vi "Cache.CheckStatus.vi"(7 "Idx":i32, 8 "error in":errorcluster, 10 "CheckStatus in":T5, 11 "Data in":T1) -> (0 "error out":errorcluster, 2 "CheckStatus out":T4, 3 "Data out":T1)   [LabVIEW 2016]
doc: "Write test results (measurement values) to proda database\n\nWabco 2017 All right reserved\nAuthor: maciej.szupienko@wabco-auto.com"
uses:
  Drivers/PLC/LowLevel/PLC.DataBlock.PLCcheckstatus.ctl
  Drivers/PLC/LowLevel/PLC.DataBlock.PCcheckstatus.ctl
  Cache.Data.ctl
  Cache.Data.Status.ctl
  Cache.Data.Sets.ctl
  Cache.ProductComponent.Data.ctl
  Tools/EventLog/EventLog.EventSource.ctl
  Tools/EventLog/EventLog.EventLevel.ctl
  Tools/Translator/Translator.Message.ctl
  Tools/EventLog/EventLog.New(array).vi
  Global/ApplicationGlobal.vi
  Tools/EventLog/EventLog.Buffer.vi
  Tools/EventLog/EventLog.File.ReadWrite.vi
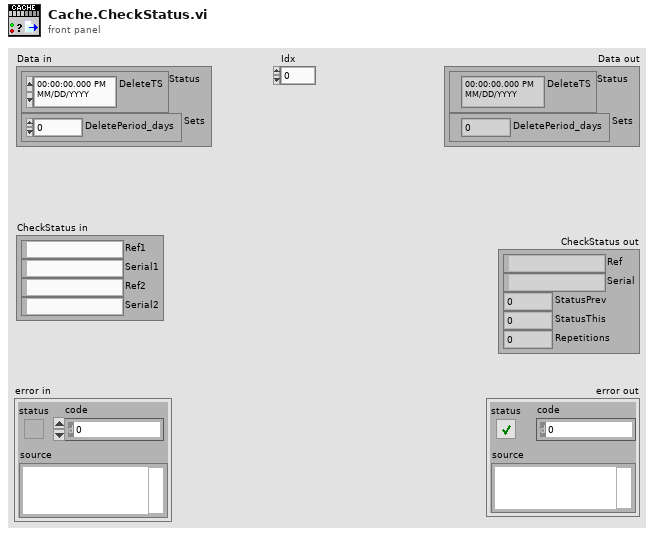
[diagram p1: front panel]
types:
  T1 = typedef "Cache.Data.ctl" = cluster{"Status":T2, "Sets":T3}
  T2 = typedef "Cache.Data.Status.ctl" = cluster{"DeleteTS":timestamp}
  T3 = typedef "Cache.Data.Sets.ctl" = cluster{"DeletePeriod_days":dbl}
  T4 = typedef "PLC.DataBlock.PCcheckstatus.ctl" = cluster{"Ref":string, "Serial":string, "StatusPrev":i8, "StatusThis":i8, "Repetitions":u8}
  T5 = typedef "PLC.DataBlock.PLCcheckstatus.ctl" = cluster{"Ref1":string, "Serial1":string, "Ref2":string, "Serial2":string}
  T6 = typedef "EventLog.EventSource.ctl" = enum16{"All", "Gui", "Cache", "PLC1", "PLC2", "PLC3", "DB", "DB01", "DB02", "DB03", "DB04", "DB05", "DB06", "DB07", "DB08", "DB09", "DB10", "DB11", "DB12", "DB13", "DB14", "DB15", "DB16"}
  T7 = typedef "Cache.ProductComponent.Data.ctl" = cluster{"Time":timestamp, "Station":string, "Ref1":string, "Serial1":string, "Ref2":string, "Serial2":string}
  T8 = typedef "Translator.Message.ctl" = enum16{"-", "Event confirmed", "Log out", "Log in", "Shutdown", "Cancel", "Start", "Continue", "Stop", "On", "Off", "OK", "NOK", "NOK %s", "This", "Prev", "Home", "Work", "In progress...", "Missing", "Empty", "Hardware failure", "Initial", "Error %d >> %s", "Error %d >> %s >> %s", "Starting %s", "Quitting %s", "Configured", "Initializing", "Quitting", "Loading", "Running %s", "Stopped", "Summary", "Do you want to continue?", "Do you want to exit?", "Log out?", "System", "All", "IDLE", "Translating...%s", "Not found", "Alarm %s", "Run", "Skip", "Abort", "Repeat", "Please wait...", "Database disconnected", "Login to database successful", "Login to database failed: %d; %s", "Get process step data for %s", "Changeover off", "Changeover into %s", "Product %s | %s found in cache with status %d at previous station", "Product %s | %s found in database with status %d at previous station", "Product %s | %s not found in cache at previous station", "Product %s | %s not found in database at previous station", "Product %s | %s found in cache with status %d at this station (%d repetion)", "Product %s | %s found in database with status %d at this station (%d repetition)", "Product %s | %s not found in cache at this station", "Product %s | %s not found in database at this station", "Product %s | %s found in cache for component %s | %s", "Product %s | %s found in database for component %s | %s", "Product not found in cache for component %s | %s", "Product not found in database for component %s | %s", "Product %s | %s connected with component %s | %s (cache)", "Product %s | %s connected with component %s | %s (database)", "New data for %s | %s (cache)", "New data for %s | %s (database)", "File %s moved (cache)", "Msg %d >> %s", "PLC LifeBit Failure", "Reconnecting DB", "Reconnecting PLC"}
  T9 = typedef "EventLog.EventLevel.ctl" = enum8{"Debug", "Info", "Warning", "Error"}
  T10 = cluster{"PrevStations":i32[], "ThisStations":i32[]}
  T11 = typedef "Cache.TestSteps.Fglb.ResultData.ctl" = cluster{"File":path, "Ref":string, "Serial":string, "Pr":T12, "PSr":T13, "TSr":cluster{"TSr":T14, "TVr":T15[]}[]}
  T12 = typedef "ProdaNG.ProcessResult.ctl" = cluster{"c_id":string, "productId":string, "processId":i32, "statusId":i32, "startTime":string, "endTime":string}
  T13 = typedef "ProdaNG.ProcessStepResult.ctl" = cluster{"c_id":string, "processResultId":string, "processStepId":i32, "statusId":i32, "operatorId":i32, "startTime":string, "endTime":string}
  T14 = typedef "ProdaNG.TestStepResult.ctl" = cluster{"c_id":string, "processStepResultId":string, "testStepId":i32, "statusId":i32}
  T15 = typedef "ProdaNG.TestValueResult.ctl" = cluster{"c_id":string, "testStepResultId":string, "testValueId":i32, "result":dbl, "statusId":i32, "contentId":string}
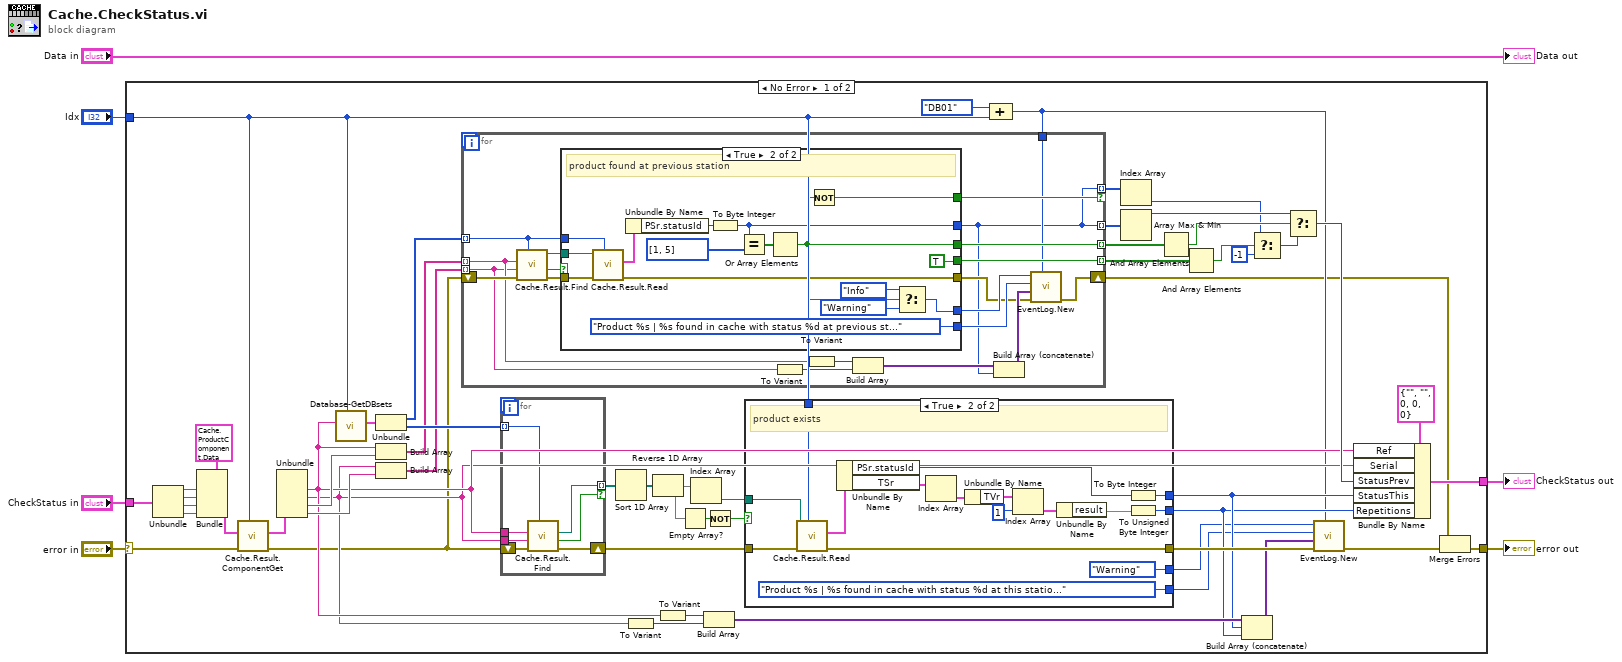
[diagram p0: block diagram]
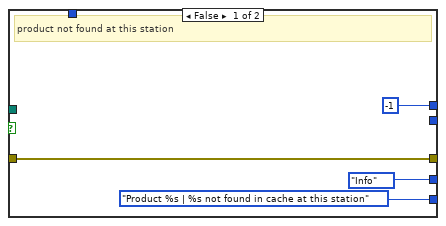
[diagram p2: hidden frame]
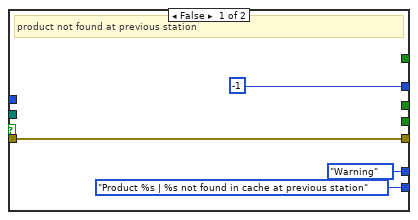
[diagram p3: hidden frame]
diagram:
  n1 = case shown="No Error" "error in" {
    selector: "error in" -> [w54 w128]
    tunnel: [w39 w128] -> w6
    tunnel: "CheckStatus in" -> [w53 _]
    tunnel: [w46 _] -> w3
    tunnel: "Idx" -> [w11 _]
    frame No Error {
      n2 = Unbundle(w53) -> ("Ref1"=w59:string, "Serial1"=w58:string, "Ref2"=w57:string, "Serial2"=w56:string)
      n3 = Bundle(cluster=T7 {"Time"=timestamp(0 s since 1904-01-01), "Station"="", "Ref1"="", "Serial1"="", "Ref2"="", "Serial2"=""} ("ProdComp in"), "Ref1"=w59, "Serial1"=w58, "Ref2"=w57, "Serial2"=w56) -> (w55:T7)  [unwired: 2 in]
      n4 = call "Cache.Result.ComponentGet.vi"("Idx"=w11, "error in (no error)"=w54, "ProdComp in"=w55) -> ("error out"=w10:errorcluster, "ProdComp out"=w9:T7)  [unwired: 6 in, 1 out]
      n5 = Unbundle(w9) -> ("Ref1"=w23:string, "Serial1"=w22:string, "Ref2"=w43:string, "Serial2"=w42:string)  [unwired: 2 out]
      n6 = call "Database-GetDBsets.vi"("Idx"=w11, "Variant"=w23) -> ("Variant Idx"=w8:T10)  [unwired: 5 in, 4 out]
      n7 = Unbundle(w8) -> ("PrevStations"=w45:i32[], "ThisStations"=w44:i32[])
      n8 = Build Array(w23, w43) -> (w41:string[])
      n9 = Build Array(w22, w42) -> (w40:string[])
      n10 = for {
        shift-right: [w66] -> w51
        shift-left: w10 -> [w67]
        tunnel: w44 -> [w65] mode=indexing
        tunnel: w23 -> [w64]
        tunnel: w22 -> [w63]
        tunnel: [w61] -> w49 mode=indexing if=w62
        n11 = call "Cache.Result.Find.vi"("Idx"=w65, "error in (no error)"=w67, "Serial"=w63, "Variant"=w64) -> ("error out"=w66:errorcluster, "Found?"=w62:bool, "File"=w61:path)  [unwired: 5 in]
      }
      n12 = Sort 1D Array(array=w49) -> (sorted array=w52:path[])
      n13 = To Variant(anything=w22) -> (Variant=w25:variant)
      n14 = Reverse 1D Array(array=w52) -> (reversed array=w48:path[])
      n15 = To Variant(anything=w23) -> (Variant=w24:variant)
      n16 = Empty Array?(array=w48) -> (empty?=w26:bool)
      n17 = Index Array(array=w48) -> (element=w7:path)  [unwired: 1 in]
      n18 = Build Array(w24, w25) -> (w20:variant[])
      n19 = Not(x=w26) -> (.not. x?=w50:bool)
      n20 = case shown="True" w50 {
        tunnel: w51 -> [w71 w87]
        tunnel: [w71 w75] -> w21
        tunnel: w7 -> [_ w86]
        tunnel: [_ w79] -> w18
        tunnel: [i8 -1 w78] -> w19
        tunnel: w11 -> [_ w76]
        tunnel: [EventLog.EventLevel."Info" ("Level (Info)") EventLog.EventLevel."Warning" ("Level (Info)")] -> w13
        tunnel: [Translator.Message."Product %s | %s not found in cache at this station" ("Message (-)") Translator.Message."Product %s | %s found in cache with status %d at this station (%d repetion)" ("Message (-)")] -> w12
        frame False {
          # "product not found at this station"
        }
        frame True {
          # "product exists"
          n21 = call "Cache.Result.Read.vi"("Idx"=w76, "error in (no error)"=w87, "ResultsPath"=w86) -> ("error out"=w75:errorcluster, "Result"=w85:T11)  [unwired: 6 in, 1 out]
          n22 = Unbundle By Name(w85) -> ("PSr.statusId"=w77:i32, "TSr"=w84:cluster{"TSr":T14, "TVr":T15[]}[])
          n23 = Index Array(array=w84) -> (element=w83:cluster{"TSr":T14, "TVr":T15[]})  [unwired: 1 in]
          n24 = Unbundle By Name(w83) -> ("TVr"=w82:T15[])
          n25 = Index Array(array=w82, index=1) -> (element=w81:T15)
          n26 = Unbundle By Name(w81) -> ("result"=w80:dbl)
          n27 = To Byte Integer(number=w77) -> (8bit integer=w78:i8)
          n28 = To Unsigned Byte Integer(number=w80) -> (unsigned 8bit integer=w79:u8)
        }
      }
      n29 = Compound Arithmetic op=ADD(EventLog.EventSource."DB01" ("Source (All)"), w11) -> (w15:i32)
      n30 = for {
        shift-right: [w94] -> w14
        shift-left: w10 -> [w107]
        tunnel: w45 -> [w88] mode=indexing
        tunnel: w41 -> [w98] mode=indexing
        tunnel: w40 -> [w97] mode=indexing
        tunnel: [w90] -> w36 mode=indexing
        tunnel: [w104] -> w37 mode=indexing
        tunnel: [w103] -> w38 mode=indexing
        tunnel: [w90] -> w30 mode=indexing if=w102
        tunnel: w15 -> [w99]
        n31 = call "Cache.Result.Find.vi"("Idx"=w88, "error in (no error)"=w107, "Serial"=w97, "Variant"=w98) -> ("error out"=w106:errorcluster, "Found?"=w89:bool, "File"=w105:path)  [unwired: 5 in]
        n32 = case shown="True" w89 {
          tunnel: w106 -> [w111 w125]
          tunnel: [w111 w124] -> w91
          tunnel: w105 -> [_ w123]
          tunnel: [i8 -1 w119] -> w90
          tunnel: [_ TRUE] -> w104
          tunnel: [_ w116] -> w103
          tunnel: [_ w118] -> w102
          tunnel: [EventLog.EventLevel."Warning" ("Level (Info)") w113] -> w93
          tunnel: [Translator.Message."Product %s | %s not found in cache at previous station" ("Message (-)") Translator.Message."Product %s | %s found in cache with status %d at previous station" ("Message (-)")] -> w92
          tunnel: w88 -> [_ w112]
          frame False {
            # "product not found at previous station"
          }
          frame True {
            # "product found at previous station"
            n33 = call "Cache.Result.Read.vi"("Idx"=w112, "error in (no error)"=w125, "ResultsPath"=w123) -> ("error out"=w124:errorcluster, "Result"=w127:T11)  [unwired: 6 in, 1 out]
            n34 = Unbundle By Name(w127) -> ("PSr.statusId"=w126:i32)
            n35 = To Byte Integer(number=w126) -> (8bit integer=w119:i8)
            n36 = Equal?(x=w119, y=i8[] [1, 5]) -> (x = y?=w121:bool[])
            n37 = Or Array Elements(Boolean array=w121) -> (logical OR=w116:bool)
            n38 = Not(x=w116) -> (.not. x?=w118:bool)
            n39 = Select(t=EventLog.EventLevel."Info" ("Level (Info)"), s=w116, f=EventLog.EventLevel."Warning" ("Level (Info)")) -> (s? t:f=w113:T9)
          }
        }
        n40 = To Variant(anything=w97) -> (Variant=w101:variant)
        n41 = To Variant(anything=w98) -> (Variant=w100:variant)
        n42 = Build Array(w100, w101) -> (w96:variant[])
        n43 = Build Array (concatenate)(w96, w90) -> (w95:variant[])
        n44 = call-poly "EventLog.New.vi"("Source (All)"=w99, "error in (no error)"=w91, "Arguments"=w95, "Message (-)"=w92, "Level (Info)"=w93) -> ("error out"=w94:errorcluster)  [unwired: 5 in, 1 out]
      }
      n45 = Index Array(array=w30) -> (element=w29:i8)  [unwired: 1 in]
      n46 = Array Max & Min(array=w36) -> (max value=w35:i8)  [unwired: 3 out]
      n47 = And Array Elements(Boolean array=w38) -> (logical AND=w34:bool)
      n48 = And Array Elements(Boolean array=w37) -> (logical AND=w33:bool)
      n49 = Build Array (concatenate)(w20, w19, w18) -> (w17:variant[])
      n50 = Select(t=w29, s=w33, f=i8 -1 ("max value")) -> (s? t:f=w31:i8)
      n51 = Select(t=w35, s=w34, f=w31) -> (s? t:f=w28:i8)
      n52 = call-poly "EventLog.New.vi"("Source (All)"=w15, "error in (no error)"=w21, "Arguments"=w17, "Message (-)"=w12, "Level (Info)"=w13) -> ("error out"=w16:errorcluster)  [unwired: 5 in, 1 out]
      n53 = Bundle By Name(cluster=T4 {"Ref"="", "Serial"="", "StatusPrev"=0, "StatusThis"=0, "Repetitions"=0} ("Data out"), "Ref"=w23, "Serial"=w22, "StatusPrev"=w28, "StatusThis"=w19, "Repetitions"=w18) -> (w46:T4)
      n54 = Merge Errors(w14, w16) -> (w39:errorcluster)
    }
    frame Error {
    }
  }
  "error out" <- w6
  "CheckStatus out" <- w3
  "Data out" <- "Data in"
